vi "Pitot-static_to_Velocity.vi"(0 "Pressure Trans voltage":dbl[](array[numeric]) format="%.2f", 1 "Stat gauge Press mmH2O  (0)":dbl format="%.1f", 2 "Atmos Press mbar  (1000)":dbl=1000.0 format="%.1f", 3 "Temp  C  (20)":dbl=20.0 format="%.1f", 4 "Pressure Trans Calib const":dbl[](array[numeric]) format="%.6f", 8 "Mano Zero":dbl) -> (5 "Velocity (m/s)":dbl[](array[numeric]) format="%.2f", 7 "Density Kg/m3":dbl format="%.2f")   [LabVIEW 2017]
doc: "this vi calculates the fluid velocity from the dynamic pressure measured with a pitot tube. Given a voltage array from the micro manometer and its calibration constants, it calculates the dynamic pressure, and knowing the temperature and absolute pressure of the fluid, calculates its velocity."
uses:
  Controls/Pressure_Units.ctl
panel:
  # "A              B"
  # "Instrument by PH. 18/2/94"
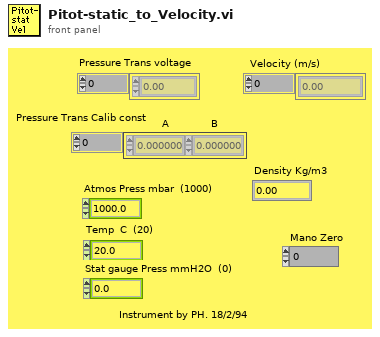
[diagram p1: front panel]
types:
  T1 = typedef "Pressure_Units.ctl" = enum16{"mmH2O", "mmHg", "Pa (N/m^2)", "mbar", "bar"}
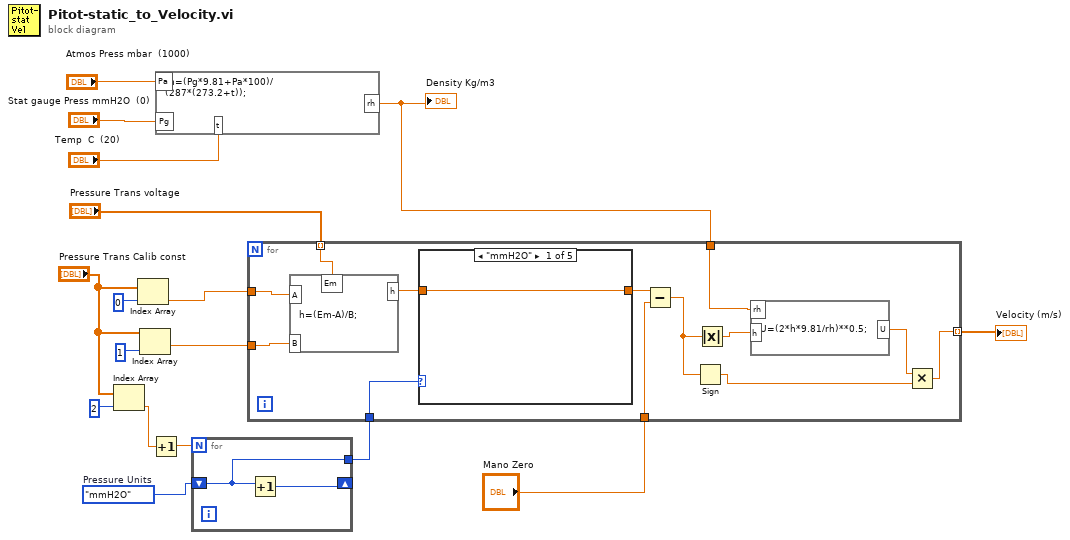
[diagram p0: block diagram]
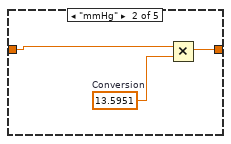
[diagram p2: hidden frame]
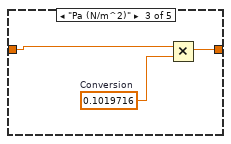
[diagram p3: hidden frame]
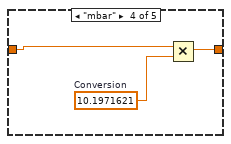
[diagram p4: hidden frame]
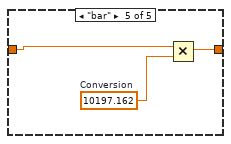
[diagram p5: hidden frame]
diagram:
  w5 = Pressure_Units."mmH2O"  # Pressure Units
  n1 = Index Array(array="Pressure Trans Calib const", index=2) -> (element=w4:dbl)
  n2 = Index Array(array="Pressure Trans Calib const", index=0) -> (element=w9:dbl)
  n3 = Index Array(array="Pressure Trans Calib const", index=1) -> (element=w8:dbl)
  n4 = Increment(x=w4) -> (x+1=w2:dbl)
  n5 = formula code="rh=(Pg*9.81+Pa*100)/\n(287*(273.2+t));"("t"="Temp  C  (20)", "Pg"="Stat gauge Press mmH2O  (0)", "Pa"="Atmos Press mbar  (1000)") -> ("rh"=w13:dbl)
  "Density Kg/m3" <- w13
  n6 = for {
    N: w2 -> [_]
    shift-right: [w19] -> _
    shift-left: w5 -> [w18]
    tunnel: [w18] -> w3
    n7 = Increment(x=w18) -> (x+1=w19:T1)
  }
  n8 = for {
    tunnel: [w25] -> w12 mode=indexing
    tunnel: w13 -> [w29]
    tunnel: "Pressure Trans voltage" -> [w30] mode=indexing
    tunnel: w8 -> [w31]
    tunnel: w9 -> [w32]
    tunnel: w3 -> [w28]
    tunnel: "Mano Zero" -> [w20]
    n9 = formula code="h=(Em-A)/B;"("Em"=w30, "B"=w31, "A"=w32) -> ("h"=w27:dbl)
    n10 = case shown="\"mmH2O\"" w28 {
      tunnel: [w33 w35 w38 w41 w44] -> w22
      tunnel: w27 -> [w33 w36 w39 w42 w45]
      frame "mmH2O" {
      }
      frame "mmHg" {
        w34 = 13.5951  # Conversion
        n11 = Multiply(x=w36, y=w34) -> (x*y=w35:dbl)
      }
      frame "Pa (N/m^2)" {
        w37 = 0.1019716  # Conversion
        n12 = Multiply(x=w39, y=w37) -> (x*y=w38:dbl)
      }
      frame "mbar" {
        w40 = 10.1971621  # Conversion
        n13 = Multiply(x=w42, y=w40) -> (x*y=w41:dbl)
      }
      frame "bar" {
        w43 = 10197.162  # Conversion
        n14 = Multiply(x=w45, y=w43) -> (x*y=w44:dbl)
      }
    }
    n15 = Subtract(x=w22, y=w20) -> (x-y=w21:dbl)
    n16 = Sign(1:w21) -> (0:w26:dbl)
    n17 = Absolute Value(x=w21) -> (abs(x)=w23:dbl)
    n18 = formula code="U=(2*h*9.81/rh)**0.5;"("rh"=w29, "h"=w23) -> ("U"=w24:dbl)
    n19 = Multiply(x=w24, y=w26) -> (x*y=w25:dbl)
  }
  "Velocity (m/s)" <- w12
